vi "阀口名称写入.vi"(4 "error in (no error)":errorcluster caption="错误输入（无错误）", 5 "Value":T3={"阀口名称自定义类型"=enum."自定义", "阀口自定义名称"={"V1"="V1", "V2"="V2", "V3"="V3", "V4"="V4", "V5"="V5", "V6"="V6", "V7"="V7", "V8"="V8", "V9"="V9", "V10"="V10", "V11"="V11", "V12"="V12", "V9-1"="V9-1", "V9-2"="V9-2", "COD慢速"="COD慢速"}} caption="值", 6 "Container State":T2 caption="容器状态", 7 "Display State In":T1={"阀口名称"={"阀口名称自定义类型"=enum."自定义", "阀口自定义名称"={"V1"="V1", "V2"="V2", "V3"="V3", "V4"="V4", "V5"="V5", "V6"="V6", "V7"="V7", "V8"="V8", "V9"="V9", "V10"="V10", "V11"="V11", "V12"="V12", "V9-1"="V9-1", "V9-2"="V9-2", "COD慢速"="V9-2"}}} caption="显示状态输入") -> (0 "error out":errorcluster caption="错误输出", 3 "Display State Out":T1={"阀口名称"={"阀口名称自定义类型"=enum."自定义", "阀口自定义名称"={"V1"="V1", "V2"="V2", "V3"="V3", "V4"="V4", "V5"="V5", "V6"="V6", "V7"="V7", "V8"="V8", "V9"="V9", "V10"="V10", "V11"="V11", "V12"="V12", "V9-1"="V9-1", "V9-2"="V9-2", "COD慢速"="V9-2"}}} caption="显示状态输出")   [LabVIEW 2016, in "调试控件V3.xctl"]
uses:
  <vilib>/_xctls/Container State.ctl
  <vilib>/_xctls/XControlSupport.lvlib
panel:
  # "将以下值显示控件替换为所需类型的显示控件。\n不要从连线板中删除该显示控件或其它显示控件。\n不要更改连线板模式。\n值显示控件应始终位于连线板输出端自顶部起第三个接线端。"
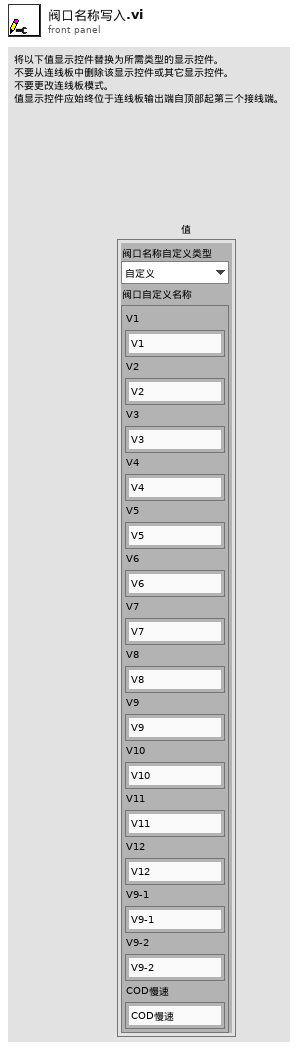
[diagram p1: front panel]
types:
  T1 = typedef "调试控件V3.xctl/状态 2.ctl" = cluster{"阀口名称":cluster{"阀口名称自定义类型":enum16{"自定义", "微站总磷总氮", "微站总磷氨氮", "微站氨氮", "固定站总磷", "固定站总氮", "固定站氨氮", "原位总磷总氮", "原位总磷氨氮", "原位总磷", "原位总氮", "原位氨氮", "原位3N1P"}, "阀口自定义名称":cluster{"V1":string, "V2":string, "V3":string, "V4":string, "V5":string, "V6":string, "V7":string, "V8":string, "V9":string, "V10":string, "V11":string, "V12":string, "V9-1":string, "V9-2":string, "COD慢速":string}}}
  T2 = typedef "XControlSupport.lvlib/Container State.ctl" = cluster{"Indicator?":bool, "Run Mode?":bool, " Refnum":refnum<vi>}
  T3 = cluster{"阀口名称自定义类型":enum16{"自定义", "微站总磷总氮", "微站总磷氨氮", "微站氨氮", "固定站总磷", "固定站总氮", "固定站氨氮", "原位总磷总氮", "原位总磷氨氮", "原位总磷", "原位总氮", "原位氨氮", "原位3N1P"}, "阀口自定义名称":cluster{"V1":string, "V2":string, "V3":string, "V4":string, "V5":string, "V6":string, "V7":string, "V8":string, "V9":string, "V10":string, "V11":string, "V12":string, "V9-1":string, "V9-2":string, "COD慢速":string}}
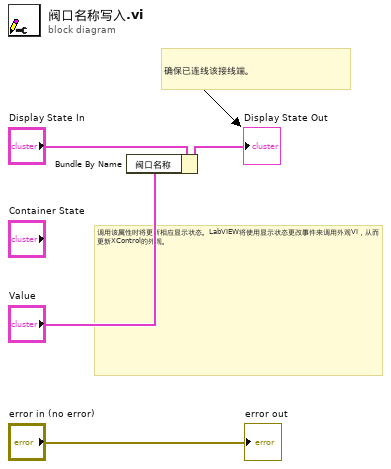
[diagram p0: block diagram]
diagram:
  # "确保已连线该接线端。"
  # "调用该属性时将更新相应显示状态。LabVIEW将使用显示状态更改事件来调用外观VI，从而更新XControl的外观。"
  n1 = Bundle By Name(cluster="Display State In", "阀口名称"="Value") -> (→"Display State Out":T1)
  "error out" <- "error in (no error)"
